vi "qTIO.vi"(0 "System no.":i32=1 min=1 max=4 step=1, 5 "error in":errorcluster) -> (14 "No. of dig. inputs":i32, 15 "No. of dig. outputs":i32, 19 "error out":errorcluster)   [LabVIEW 2020]
doc: "Returns the number of digital inputs and outputs available in the controller. \n\nE-761: The E-761 has no genuine digital input and output lines, but the analog input is internally interpreted as digital input for triggering tasks (see E-761 user manual), and its signal state can be queried by DIO?vi."
panel:
  # "Returns the number of digital inputs and outputs available \nin the controller."
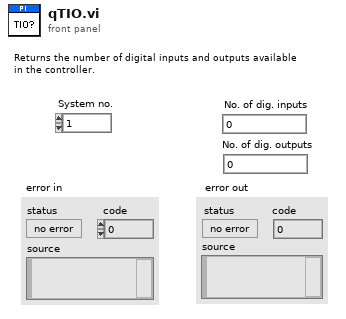
[diagram p1: front panel]
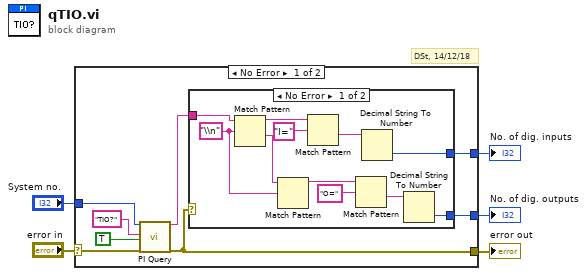
[diagram p0: block diagram]
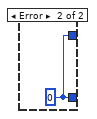
[diagram p2: hidden frame]
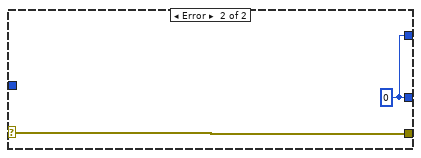
[diagram p3: hidden frame]
diagram:
  # "DSt, 14/12/18"
  n1 = case shown="No Error" "error in" {
    selector: "error in" -> [w8 w27]
    tunnel: [w13 w26] -> w5
    tunnel: "System no." -> [w11 _]
    tunnel: [w9 w26] -> w3
    tunnel: [w6 w27] -> w2
    frame No Error {
      n2 = call "PI Query.vi"("System no."=w11, "String to send"="TIO?", "Attach termination char.?"=TRUE ("Attach Linefeed?"), "error in"=w8) -> ("String read"=w7:string, "error out"=w6:errorcluster)  [unwired: 3 in, 11 out]
      n3 = case shown="No Error" w6 {
        tunnel: w7 -> [w24 _]
        tunnel: [w22 w25] -> w13
        tunnel: [w23 w25] -> w9
        frame No Error {
          w14 = "\\n" ("regular expression")
          n4 = Match Pattern(string=w24, regular expression=w14) -> (before substring=w18:string, after substring=w21:string)  [unwired: 3 out]
          n5 = Match Pattern(string=w21, regular expression=w14) -> (before substring=w15:string)  [unwired: 4 out]
          n6 = Match Pattern(string=w18, regular expression="I=") -> (after substring=w19:string)  [unwired: 4 out]
          n7 = Match Pattern(string=w15, regular expression="O=") -> (after substring=w16:string)  [unwired: 4 out]
          n8 = Decimal String To Number(string=w19) -> (number=w22:i32)  [unwired: 3 out]
          n9 = Decimal String To Number(string=w16) -> (number=w23:i32)  [unwired: 3 out]
        }
        frame Error {
          w25 = 0
        }
      }
    }
    frame Error {
      w26 = 0
    }
  }
  "error out" <- w2
  "No. of dig. inputs" <- w5
  "No. of dig. outputs" <- w3
